vi "Image_Handler_2.0.vi"(0 "Camera":T5, 5 "Data":T1={"Camera 1"={"Camera1"="", "Cam 1"=FALSE, "CAM1 Model"=enum."a2A5328-15ucBAS", "Cam1 ID"=0}, "Camera 2"={"Camera2"="", "Cam 2"=FALSE, "CAM2 Model"=enum."a2A5328-15ucBAS", "Cam2 ID"=0}, "Image"={"Camera1_Img"=refnum, "Camera2_Img"=refnum, "Img1_Orig_Disp"=refnum, "Img2_Orig_Disp"=refnum, "Img1_Orig_RGB"=refnum, "Img2_Orig_RGB"=refnum, "Blue_Plane_Extract"=refnum, "Subtracted_Plane"=refnum, "Img1_Binary"=refnum, "Img2_Binary"=refnum, "Crop_Mask"=refnum, "Img1_Save"=refnum, "Img2_Save"=refnum, "Img1_Cali_Full"=refnum, "Img2_Cali_Full"=refnum, "Img1_Cali_Detect"=refnum, "Img2_Cali_Detect"=refnum}, "Ques"={"Cam 1 queue"=refnum, "Cam 2 queue"=refnum, "Cam 1 - save queue"=refnum, "Cam 2 - save queue"=refnum, "Image Process Queue Size"=500, "Image Save Queue Size"=500, "Overload threshold"=500, "Max large object threshold"=0}, "Arduino SRS"={"Pinch-valve"="", "Actuator"=FALSE, "Open(T)/Close(F)"=FALSE, "Arduino Uno"=""}, "Pump"={"Port"="", "Connection"=FALSE, "Pump State"=FALSE, "Pump Model"=enum."XLP6000", "Pump size"=FALSE, "Flush Size"=0, "Dispense Speed"=100, "Command"="", "Pump"=""}, "Camera settings"={"Detection settings"={"Sample size threshold"=500, "Detection Region %"=30.0, "Timeout Sample"=200}, "Lens/camera settings"={"Aperture"=enum."Item 0", "Legacy Cam Attributes"=FALSE, "Max Framerate"=100, "Exposure Time"=1000.0, "Framerate"=15}, "Crop settings"={"Cam1"={"Rectangle 1"={"Left"=0, "Top"=0, "Right"=0, "Bottom"=0, "Rotation"=0.0}, "Camera Orientation 1"="", "Pixel to mm 1"=0.0}, "Cam2"={"Rectangle 2"={"Left"=0, "Top"=0, "Right"=0, "Bottom"=0, "Rotation"=0.0}, "Camera Orientation 2"="", "Pixel to mm 2"=0.0}}}, "Arduino ISS"={"Mega F3"="", "Phase3"=FALSE, "Barcode"="", "Sorting sys."=FALSE, "Initial size"=0.0, "Size Interval"=0.0, "Mun. of containers"=0.0, "Container nr."=0.0, "Arduino Mega"=""}, "Img_Capt"=FALSE, "Empty_Refill"=FALSE, "I don't think is in use"={"Light intensity"=100}, "Extended setup"={"Location"="Station", "Latitude"="Station", "Longitude"="Station", "Determiner"="Station", "Sex"="Station", "Station"="", "Collection date"=""}, "Main interface"={"Sample Name"="Test Sample", "Operator"="JFR", "Species Name"="", "Other Notes"=""}, "Tap1"=0, "SystemVersion"=0, "System Serial"="", "Exit"=FALSE, "Kuvette Full"=FALSE, "Core JKI"={"Current VI Reference"=refnum, "Close Panel on Exit?"=FALSE}, "Calibration"={"Calibration 1"=path "C:/Users/au540322/Desktop/IHS_Project/images/Debris/Debris_0/Debris_0_2019_06_01-23-32-49-686.PNG", "Calibration 2"=path "C:/Users/au540322/Desktop/IHS_Project/images/Debris/Debris_0/Debris_0_2019_06_01-23-32-49-686.PNG", "Detect 1"=path "C:/Users/au540322/Desktop/IHS_Project/images/Debris/Debris_0/Debris_0_2019_06_01-23-32-49-686.PNG", "Detect 2"=path "C:/Users/au540322/Desktop/IHS_Project/images/Debris/Debris_0/Debris_0_2019_06_01-23-32-49-686.PNG"}, "Flush Insect"=FALSE, "Auto Flush"=FALSE} {"SystemVersion" items=["Standard", "XL"]; "Tap1" items=["Session Data", "Extended Setup", "Buffer", "Camera", "Dispenser", "Stats", "Connections"]; "I don't think is in use"."Light intensity" scale=0.0..100.0; "Camera settings"."Crop settings"."Cam2"."Rectangle 2"."Rotation" format="%.2f"; "Camera settings"."Crop settings"."Cam2"."Rectangle 2"."Left" scale=0.0..1024.0; "Camera settings"."Crop settings"."Cam2"."Rectangle 2"."Right" scale=0.0..1024.0; "Camera settings"."Crop settings"."Cam1"."Rectangle 1"."Rotation" format="%.2f"; "Camera settings"."Crop settings"."Cam1"."Rectangle 1"."Left" scale=0.0..1024.0; "Camera settings"."Crop settings"."Cam1"."Rectangle 1"."Right" scale=0.0..1024.0; "Camera settings"."Lens/camera settings"."Framerate" min=1; "Camera settings"."Lens/camera settings"."Max Framerate" min=1; "Camera settings"."Detection settings"."Sample size threshold" min=1; "Pump"."Dispense Speed" min=1; "Pump"."Flush Size" min=0 max=6000 step=100; "Ques"."Overload threshold" min=1; "Ques"."Image Save Queue Size" min=1; "Ques"."Image Process Queue Size" min=1}, 9 "Prev. sample":i32, 11 "Timeout in":i32) -> (2 "Detection error":errorcluster, 3 "Object":bool, 4 "Detected object":T3, 6 "Image Out":T3, 8 "Binary":T3, 10 "Sample nr":i32, 15 "Timeout out":i32)   [LabVIEW 2024]
uses:
  Camera_ID.ctl
  <vilib>/vision/Image Controls.llb/IMAQ Image.ctl
  controls/Data_JKI.ctl
  <vilib>/userDefined/High Color/IMAQdx.ctl
panel:
  out "error out 1":errorcluster
  out "error out 2":errorcluster
  in  "error in":errorcluster
  out "error out":errorcluster
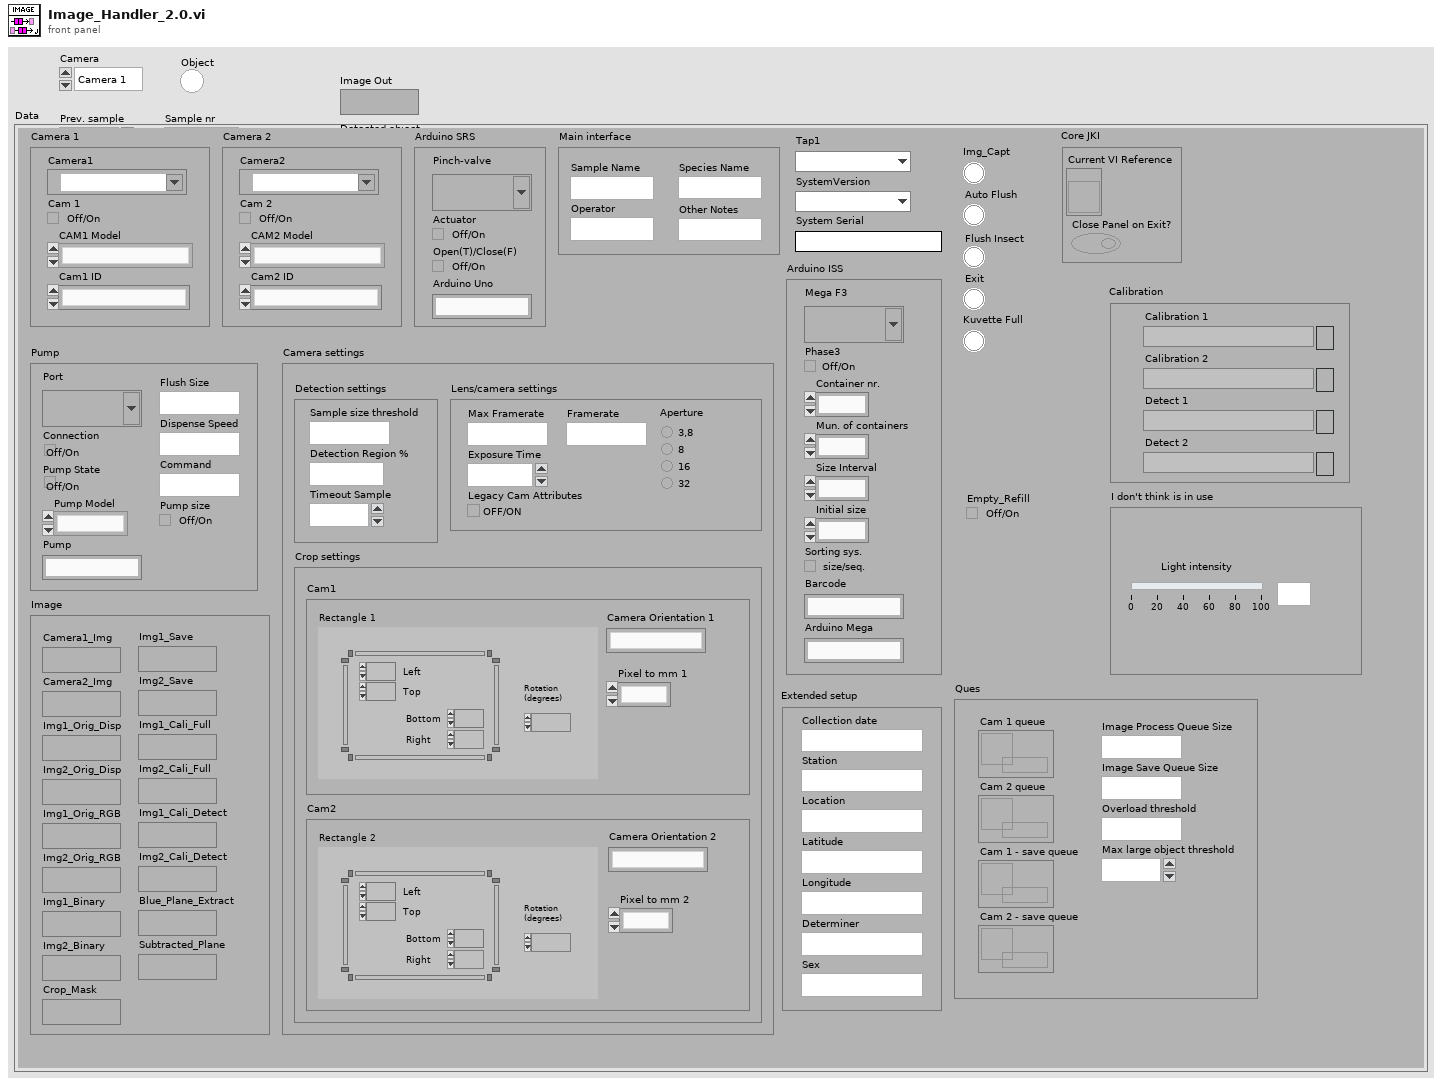
[diagram p1: front panel]
types:
  T1 = typedef "Data_JKI.ctl" = cluster{"Camera 1":cluster{"Camera1":T2, "Cam 1":bool, "CAM1 Model":enum16{"a2A5328-15ucBAS", "acA1920-155uc"}, "Cam1 ID":i32}, "Camera 2":cluster{"Camera2":T2, "Cam 2":bool, "CAM2 Model":enum16{"a2A5328-15ucBAS", "acA1920-155uc"}, "Cam2 ID":i32}, "Image":cluster{"Camera1_Img":T3, "Camera2_Img":T3, "Img1_Orig_Disp":T3, "Img2_Orig_Disp":T3, "Img1_Orig_RGB":T3, "Img2_Orig_RGB":T3, "Blue_Plane_Extract":T3, "Subtracted_Plane":T3, "Img1_Binary":T3, "Img2_Binary":T3, "Crop_Mask":T3, "Img1_Save":T3, "Img2_Save":T3, "Img1_Cali_Full":T3, "Img2_Cali_Full":T3, "Img1_Cali_Detect":T3, "Img2_Cali_Detect":T3}, "Ques":cluster{"Cam 1 queue":refnum<queue>, "Cam 2 queue":refnum<queue>, "Cam 1 - save queue":refnum<queue>, "Cam 2 - save queue":refnum<queue>, "Image Process Queue Size":i32, "Image Save Queue Size":i32, "Overload threshold":i32, "Max large object threshold":i32}, "Arduino SRS":cluster{"Pinch-valve":refnum<visa-resource-name>, "Actuator":bool, "Open(T)/Close(F)":bool, "Arduino Uno":string}, "Pump":cluster{"Port":refnum<visa-resource-name>, "Connection":bool, "Pump State":bool, "Pump Model":enum16{"XLP6000", "XL1000"}, "Pump size":bool, "Flush Size":i32, "Dispense Speed":i32, "Command":string, "Pump":string}, "Camera settings":cluster{"Detection settings":cluster{"Sample size threshold":i32, "Detection Region %":dbl, "Timeout Sample":i32}, "Lens/camera settings":cluster{"Aperture":enum32{"Item 0", "Item 1", "Item 2", "Item 3"}, "Legacy Cam Attributes":bool, "Max Framerate":i32, "Exposure Time":dbl, "Framerate":i32}, "Crop settings":cluster{"Cam1":cluster{"Rectangle 1":T4, "Camera Orientation 1":string, "Pixel to mm 1":dbl}, "Cam2":cluster{"Rectangle 2":T4, "Camera Orientation 2":string, "Pixel to mm 2":dbl}}}, "Arduino ISS":cluster{"Mega F3":refnum<visa-resource-name>, "Phase3":bool, "Barcode":string, "Sorting sys.":bool, "Initial size":dbl, "Size Interval":dbl, "Mun. of containers":dbl, "Container nr.":dbl, "Arduino Mega":string}, "Img_Capt":bool, "Empty_Refill":bool, "I don't think is in use":cluster{"Light intensity":i32}, "Extended setup":cluster{"Location":string, "Latitude":string, "Longitude":string, "Determiner":string, "Sex":string, "Station":string, "Collection date":string}, "Main interface":cluster{"Sample Name":string, "Operator":string, "Species Name":string, "Other Notes":string}, "Tap1":u16, "SystemVersion":u16, "System Serial":string, "Exit":bool, "Kuvette Full":bool, "Core JKI":cluster{"Current VI Reference":refnum<vi>, "Close Panel on Exit?":bool}, "Calibration":cluster{"Calibration 1":path, "Calibration 2":path, "Detect 1":path, "Detect 2":path}, "Flush Insect":bool, "Auto Flush":bool}
  T2 = typedef "IMAQdx.ctl" = refnum<k21>
  T3 = typedef "IMAQ Image.ctl" = refnum<image>
  T4 = typedef "IMAQ Rectangle" = cluster{"Left":i32, "Top":i32, "Right":i32, "Bottom":i32, "Rotation":dbl}
  T5 = typedef "Camera_ID.ctl" = enum16{"Camera 1", "Camera 2"}
  T6 = cluster{"Image Pixels (U32)":u32[][], "Detect Movement":bool, "Timestamp_snap":string}
  T7 = cluster{"Global Rectangle":i32[], "Contours":cluster{"ID":enum32{"External", "Internal"}, "Type":u32, "Coordinates":i32[]}[]}
  T8 = cluster{"result string":string, "Image Pixels (U32)":u32[][], "Prev. sample":i32, "Sample Data":dbl[], "ROI descriptor":cluster{"Global Rectangle":i32[], "Contours":cluster{"ID":enum32{"External", "Internal"}, "Type":u32, "Coordinates":i32[]}[]}}
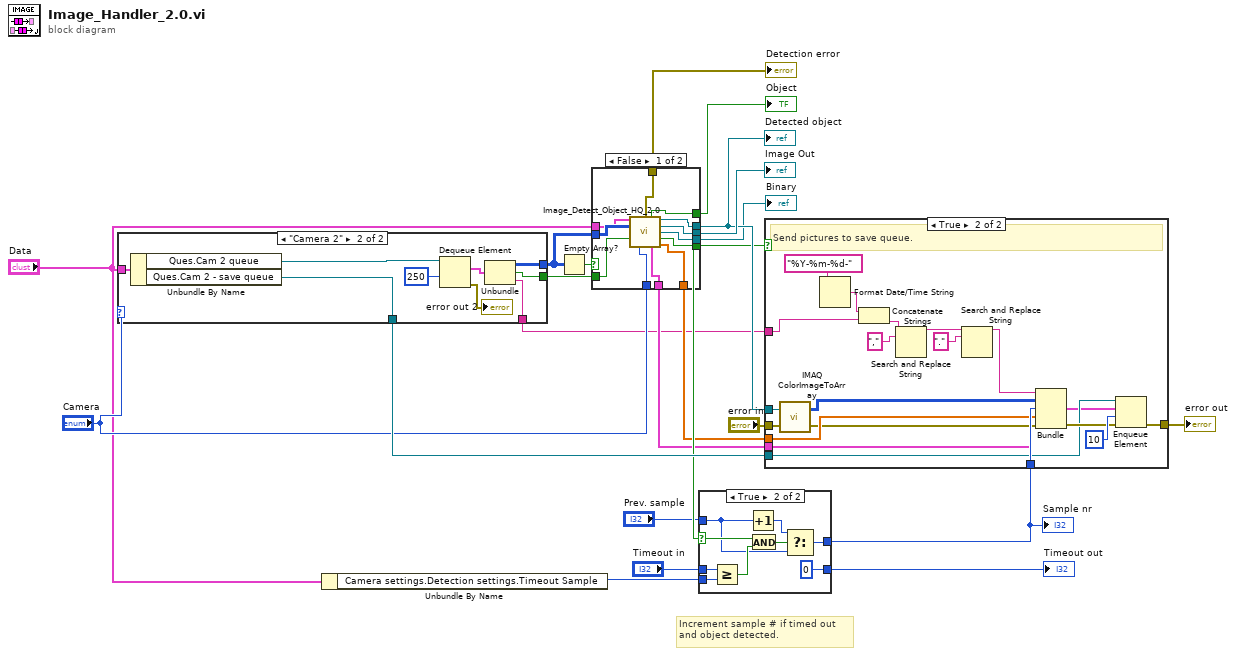
[diagram p0: block diagram]
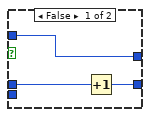
[diagram p2: hidden frame]
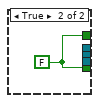
[diagram p4: hidden frame]
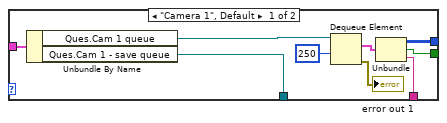
[diagram p5: hidden frame]
diagram:
  # "Increment sample # if timed out \nand object detected."
  n1 = case shown="\"Camera 2\"" "Camera" {
    tunnel: "Data" -> [w31 w40]
    tunnel: [w28 w36] -> w19
    tunnel: [w27 w35] -> w11
    tunnel: [w26 w34] -> w7
    tunnel: [w23 w32] -> w2
    frame "Camera 1", Default {
      n2 = Unbundle By Name(w31) -> ("Ques.Cam 1 queue"=w24:refnum<queue>, "Ques.Cam 1 - save queue"=w28:refnum<queue>)
      n3 = Dequeue Element(queue=w24, timeout in ms (-1)=250) -> (element=w25:T6, error out=→"error out 1":errorcluster)  [unwired: 1 in, 2 out]
      n4 = Unbundle(w25) -> ("Image Pixels (U32)"=w27:u32[][], "Detect Movement"=w26:bool, "Timestamp_snap"=w23:string)
    }
    frame "Camera 2" {
      n5 = Unbundle By Name(w40) -> ("Ques.Cam 2 queue"=w33:refnum<queue>, "Ques.Cam 2 - save queue"=w36:refnum<queue>)
      n6 = Dequeue Element(queue=w33, timeout in ms (-1)=250) -> (element=w38:T6, error out=→"error out 2":errorcluster)  [unwired: 1 in, 2 out]
      n7 = Unbundle(w38) -> ("Image Pixels (U32)"=w35:u32[][], "Detect Movement"=w34:bool, "Timestamp_snap"=w32:string)
    }
  }
  n8 = Unbundle By Name("Data") -> ("Camera settings.Detection settings.Timeout Sample"=w13:i32)
  n9 = Empty Array?(array=w11) -> (empty?=w22:bool)
  n10 = case shown="False" w22 {
    tunnel: [w43 _] -> w20
    tunnel: [w46 w53] -> w15
    tunnel: "Data" -> [w50 _]
    tunnel: "Camera" -> [w49 _]
    tunnel: [w44 _] -> w21
    tunnel: w11 -> [w51 _]
    tunnel: [w42 w53] -> w8
    tunnel: w7 -> [w52 _]
    tunnel: [w47 _] -> w6
    tunnel: [w45 _] -> w5
    tunnel: [w48 _] -> w4
    tunnel: [w41 _] -> w3
    frame False {
      n11 = call "Image_Detect_Object_HQ_2.0.vi"("Data"=w50, "Image Pixels (U32)"=w51, "Detect Crop"=w52, "Camera"=w49) -> ("error out"=w41:errorcluster, "Obj Size"=w42:bool, "Detected object"=w43:T3, "Image Out"=w44:T3, "Binary"=w45:T3, "Object Accept"=w46:bool, "ROI descriptor"=w48:T7, "Sample Data"=w47:dbl[])  [unwired: 4 in]
    }
    frame True {
      w53 = FALSE ("Object detected")
    }
  }
  "Detected object" <- w20
  "Image Out" <- w21
  "Binary" <- w5
  "Object" <- w8
  "Detection error" <- w3
  n12 = case shown="True" w15 {
    selector: w15 -> [_ w65]
    tunnel: w13 -> [_ w64]
    tunnel: [w56 0] -> w14
    tunnel: [w55 w59] -> w12
    tunnel: "Prev. sample" -> [w55 w58]
    tunnel: "Timeout in" -> [w54 w57]
    frame False {
      n13 = Increment(x=w54) -> (x+1=w56:i32)
    }
    frame True {
      n14 = Greater Or Equal?(x=w57, y=w64) -> (x >= y?=w63:bool)
      n15 = Increment(x=w58) -> (x+1=w60:i32)
      n16 = And(x=w65, y=w63) -> (x .and. y?=w61:bool)
      n17 = Select(t=w60, s=w61, f=w58) -> (s? t:f=w59:i32)
    }
  }
  "Sample nr" <- w12
  "Timeout out" <- w14
  n18 = case shown="True" w15 {
    tunnel: w20 -> [_ w81]
    tunnel: w19 -> [_ w77]
    tunnel: "error in" -> [w66 w80]
    tunnel: [w66 w85] -> w16
    tunnel: w12 -> [_ w84]
    tunnel: w6 -> [_ w82]
    tunnel: w4 -> [_ w76]
    tunnel: w2 -> [_ w72]
    frame False {
      # "No object within criteria."
    }
    frame True {
      # "Send pictures to save queue."
      n19 = call "IMAQ ColorImageToArray"("Image"=w81, "error in (no error)"=w80) -> ("Image Pixels (U32)"=w78:u32[][], "error out"=w79:errorcluster)  [unwired: 2 in, 1 out]
      n20 = Format Date/Time String(time format string (%c)="%Y-%m-%d-") -> (date/time string=w74:string)  [unwired: 2 in]
      n21 = Concatenate Strings(w74, w72) -> (w68:string)
      n22 = Search and Replace String(input string=w68, search string=",") -> (result string=w69:string)  [unwired: 6 in, 3 out]
      n23 = Search and Replace String(input string=w69, search string=".") -> (result string=w67:string)  [unwired: 6 in, 3 out]
      n24 = Bundle("result string"=w67, "Image Pixels (U32)"=w78, "Prev. sample"=w84, "Sample Data"=w82, "ROI descriptor"=w76) -> (w75:T8)  [unwired: 1 in]
      n25 = Enqueue Element(queue=w77, element=w75, timeout in ms (-1)=10, error in (no error)=w79) -> (error out=w85:errorcluster)  [unwired: 2 out]
    }
  }
  "error out" <- w16
